vi "SQLite Add Subcategory Test.vi"(7 "Test DB Set Up Command":string, 8 "Error In (no error)":errorcluster, 11 "SQLite DB Operator In":refnum<class "SQLite DB Operator.lvclass">) -> (0 "Error Out":errorcluster, 3 "SQLite DB Operator Out":refnum<class "SQLite DB Operator.lvclass">)   [LabVIEW 2023]
uses:
  SQLite DB Operator/SQLite DB Operator.lvclass
  DB Records/Expenses Tracker Record/Public/Ctrls/Subcategory.ctl
  DB Records/Expenses Tracker Subcategory/Expenses Tracker Subcategory.lvclass
  H:/Desktop/LabVIEW/LabView Repo/Expenses-Tracker-DB-Operator/DB Records/Expenses Tracker Record/Expenses Tracker Record.lvclass
  <vilib>/drjdpowell/SQLite Library/SQL Connection/Execute SQL (1D Cluster).vi
  <vilib>/addons/_JKI Toolkits/Caraya/classes/Test/Test.lvclass
  <vilib>/drjdpowell/SQLite Library/SQLite.lvlib
  DB Records/Expenses Tracker Record/Expenses Tracker Record.lvclass
  <vilib>/drjdpowell/SQLite Library/SQL Connection/Connection.lvclass
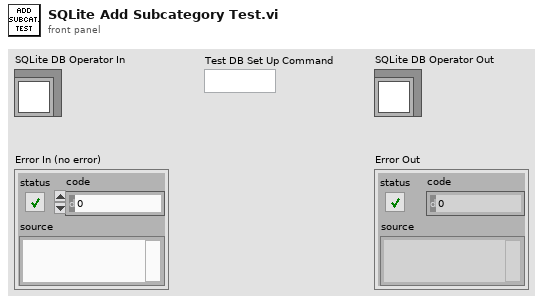
[diagram p1: front panel]
types:
  T1 = typedef "Expenses Tracker Record.lvclass/Subcategory.ctl" = cluster{"ID":u32, "Name":string, "Category":u32}
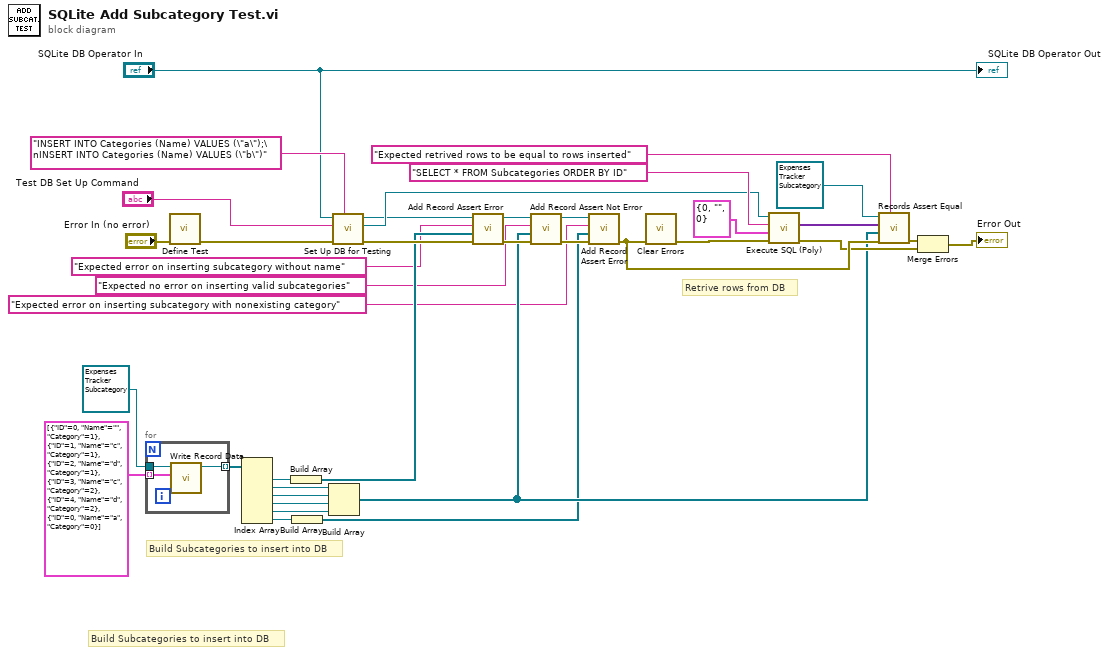
[diagram p0: block diagram]
diagram:
  # "Retrive rows from DB"
  # "Build Subcategories to insert into DB"
  # "Build Subcategories to insert into DB"
  n1 = for {
    tunnel: T1[] [{"ID"=0, "Name"="", "Category"=1}, {"ID"=1, "Name"="c", "Category"=1}, {"ID"=2, "Name"="d", "Category"=1}, {"ID"=3, "Name"="c", "Category"=2}, {"ID"=4, "Name"="d", "Category"=2}, {"ID"=0, "Name"="a", "Category"=0}] ("Array") -> [w40] mode=indexing
    tunnel: refnum<class "Expenses Tracker Subcategory.lvclass"> refnum ("Expenses Tracker Category") -> [w39]
    tunnel: [w38] -> w34 mode=indexing
    n2 = call-dynamic "Write Record Data.vi"("Record"=w40, "Expenses Tracker Subcategory In"=w39) -> ("Expenses Tracker Subcategory Out"=w38:refnum<class "Expenses Tracker Subcategory.lvclass">)  [unwired: 8 in, 1 out]
  }
  n3 = call <vilib>:"Define Test.vi"("error in (no error)"="Error In (no error)") -> ("error out"=w24:errorcluster)  [unwired: 9 in, 1 out]
  n4 = Index Array(array=w34) -> (element #1=w33:refnum<class "Expenses Tracker Subcategory.lvclass">, element #2=w32:refnum<class "Expenses Tracker Subcategory.lvclass">, element #3=w31:refnum<class "Expenses Tracker Subcategory.lvclass">, element #4=w28:refnum<class "Expenses Tracker Subcategory.lvclass">, element #5=w27:refnum<class "Expenses Tracker Subcategory.lvclass">, element #6=w2:refnum<class "Expenses Tracker Subcategory.lvclass">)  [unwired: 6 in]
  n5 = Build Array(w33) -> (w12:refnum<class "Expenses Tracker Subcategory.lvclass">[])
  n6 = Build Array(w2) -> (w1:refnum<class "Expenses Tracker Subcategory.lvclass">[])
  n7 = Build Array(w32, w31, w28, w27) -> (w4:refnum<class "Expenses Tracker Subcategory.lvclass">[])
  n8 = call "Set Up DB for Testing.vi"("Additional Set Up Commands"="INSERT INTO Categories (Name) VALUES (\"a\");\nINSERT INTO Categories (Name) VALUES (\"b\")", "Error In (no error)"=w24, "Test DB Set Up Command"="Test DB Set Up Command", "SQLite DB Operator In"="SQLite DB Operator In") -> ("Error Out"=w13:errorcluster, "SQLite Connection"=w26:refnum<class "Connection.lvclass">, "SQLite DB Operator Out"=w11:refnum<class "SQLite DB Operator.lvclass">)  [unwired: 5 in]
  n9 = call "Add Record Assert Error.vi"("Error In"=w13, "Records"=w12, "Assertion Label"="Expected error on inserting subcategory without name" ("Label (VI Title)"), "SQLite DB Operator In"=w11) -> ("Error Out"=w16:errorcluster, "SQLite DB Operator Out"=w17:refnum<class "SQLite DB Operator.lvclass">)  [unwired: 6 in]
  n10 = call "Add Record Assert Not Error.vi"("Error In"=w16, "Records"=w4, "Assertion Label"="Expected no error on inserting valid subcategories" ("Label (VI Title)"), "SQLite DB Operator In"=w17) -> ("Error Out"=w14:errorcluster, "SQLite DB Operator Out"=w15:refnum<class "SQLite DB Operator.lvclass">)  [unwired: 6 in]
  n11 = call "Add Record Assert Error.vi"("Error In"=w14, "Records"=w1, "Assertion Label"="Expected error on inserting subcategory with nonexisting category" ("Label (VI Title)"), "SQLite DB Operator In"=w15) -> ("Error Out"=w9:errorcluster)  [unwired: 6 in, 1 out]
  n12 = call <vilib>:"Clear Errors.vi"("error in (no error)"=w9) -> ("error out"=w21:errorcluster)  [unwired: 5 in, 1 out]
  n13 = call-poly <vilib>:"Execute SQL (Poly).vi"("error in (no error)"=w21, "Cluster (or Array of Clusters)"=T1 {"ID"=0, "Name"="", "Category"=0} ("Subcategory"), "SQL"="SELECT * FROM Subcategories ORDER BY ID", "SQLite Connection in"=w26) -> ("error out"=w7:errorcluster, "Result Set (Array of Clusters)"=w20:variant[])  [unwired: 5 in, 1 out]
  n14 = call "Records Assert Equal.vi"("Assertion Label"="Expected retrived rows to be equal to rows inserted" ("Label (VI Title)"), "Error In"=w9, "Correct Records"=w4, "Typedef Records"=w20, "Expenses Tracker Record In"=refnum<class "Expenses Tracker Subcategory.lvclass"> refnum ("Expenses Tracker Category")) -> ("Error Out"=w8:errorcluster)  [unwired: 6 in]
  n15 = Merge Errors(w8, w7) -> (→"Error Out":errorcluster)
  "SQLite DB Operator Out" <- "SQLite DB Operator In"
